vi "Create DVR_Queue.vi"(11 "error in (no error)":errorcluster) -> (4 "Queue DVR out":refnum<data-value>, 15 "error out":errorcluster)   [LabVIEW 2020, in "Data Communication Transmitter.lvlib" / "Queue.lvclass"]
doc: "This VI is used to create DVR for queue to transfer the data cluster"
uses:
  Classes/Children/Intra-Application/Children/With Data/Children/Queues/Queue.lvclass
  Classes/Children/Intra-Application/Children/With Data/Children/Queues/Queue.lvclass/Queue.ctl
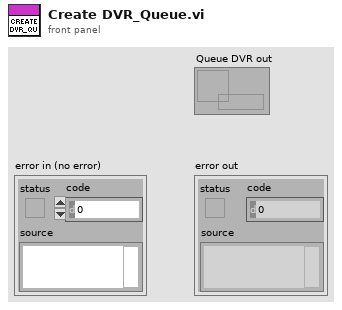
[diagram p1: front panel]
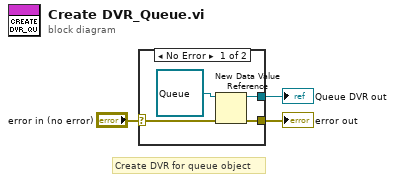
[diagram p0: block diagram]
diagram:
  # "Create DVR for queue object"
  n1 = case shown="No Error" "error in (no error)" {
    selector: "error in (no error)" -> [w7 w8]
    tunnel: [w6 w8] -> w2
    tunnel: [w4 _] -> w1
    frame No Error {
      n2 = New Data Value Reference(data value=refnum<class "Queue.lvclass"> refnum ("Queue in"), error in=w7) -> (data value reference=w4:refnum<data-value>, error out=w6:errorcluster)
    }
    frame Error {
    }
  }
  "error out" <- w2
  "Queue DVR out" <- w1
